vi "Basic test.vi"() -> ()   [LabVIEW 2018]
uses:
  <vilib>/FPGAPlugInAG/cRIO-9074/niLvFpga_Open_cRIO-9074.vi
  <vilib>/Utility/error.llb/Error Cluster From Error Code.vi
  <vilib>/rvi/errors/niLvFpgaAdjustHostInterfaceError.vi
  <vilib>/FPGAPlugInAG/cRIO-9074/niLvFpga_Close_cRIO-9074.vi
  <vilib>/rvi/interface/nirviOpenFPGA/nirviOpenFPGA.xnode
  FPGA Bitfiles/NewCompressorRig_FPGATarget_FPGAMain_dxecnm0rUT0.lvbitx
  FPGA/FPGA Main.vi
  <vilib>/rvi/interface/nirviReadWriteControl/nirviReadWriteControl.xnode
  <vilib>/rvi/interface/nirviCloseFPGA/nirviCloseFPGA.xnode
  NiFpgaLv.dll
panel:
  in  "Start":bool
  out "loop period (usec)":u32
  out "error out":errorcluster
  out "Acquiring?":bool
  in  "Stop":bool
  in  "Stop":bool
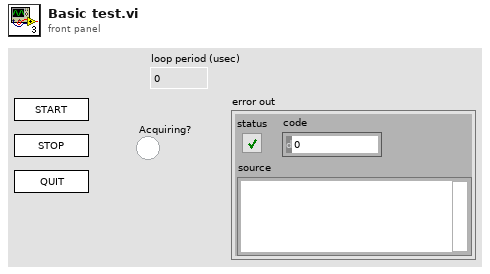
[diagram p1: front panel]
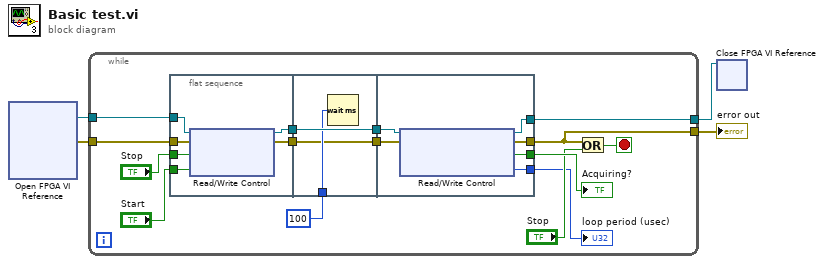
[diagram p0: block diagram]
diagram:
  n1 = xnode "Open FPGA VI Reference"() -> ("FPGA VI Reference Out"=w3:refnum<k20>, "error out"=w2:errorcluster)  [unwired: 2 in]
  n2 = while {
    tunnel: w3 -> [w18]
    tunnel: [w15] -> w4
    tunnel: w2 -> [w12]
    tunnel: [w7] -> w1
    stop <- w8 stop-if-true
    n3 = flat-sequence {
      tunnel: "Stop" -> [w25]
      tunnel: w18 -> [w24]
      tunnel: [w23] -> w17
      tunnel: w12 -> [w22]
      tunnel: [w21] -> w10
      tunnel: "Start" -> [w20]
      tunnel: w17 -> [w28]
      tunnel: [w28] -> w16
      tunnel: u32 100 ("milliseconds to wait") -> [w27]
      tunnel: [w26] -> w11
      tunnel: w10 -> [w26]
      tunnel: w16 -> [w34]
      tunnel: [w33] -> w15
      tunnel: [w32] -> w14
      tunnel: w11 -> [w31]
      tunnel: [w30] -> w7
      tunnel: [w29] -> w6
      frame #0 {
        n4 = xnode "Read/Write Control"("FPGA VI Reference In"=w24, "error in"=w22, "Stop acquire"=w25, "Start acquire"=w20) -> ("FPGA VI Reference Out"=w23:refnum<k20>, "error out"=w21:errorcluster)
      }
      frame #1 {
        n5 = Wait (ms)(milliseconds to wait=w27) -> ()  [unwired: 1 out]
      }
      frame #2 {
        n6 = xnode "Read/Write Control"("FPGA VI Reference In"=w34, "error in"=w31) -> ("FPGA VI Reference Out"=w33:refnum<k20>, "error out"=w30:errorcluster, "Start acquire"=w32:bool, "loop period (usec)"=w29:u32)
      }
    }
    n7 = Or(x=w7, y="Stop") -> (x .or. y?=w8:bool)
    "Acquiring?" <- w14
    "loop period (usec)" <- w6
  }
  "error out" <- w1
  n8 = xnode "Close FPGA VI Reference"("FPGA VI Reference In"=w4) -> ()  [unwired: 1 in, 1 out]
